vi "Read Value.vi"(8 "error in (no error)":errorcluster, 11 "Float D Element in":refnum<class "Float D Element.lvclass">) -> (0 "error out":errorcluster, 2 "Value":sgl, 3 "Float D Element out":refnum<class "Float D Element.lvclass">)   [LabVIEW 2018, in "D Datagrid Library.lvlib" / "Float D Element.lvclass"]
uses:
  Float D Element.lvclass
  Float D Element.lvclass/Float D Element.ctl
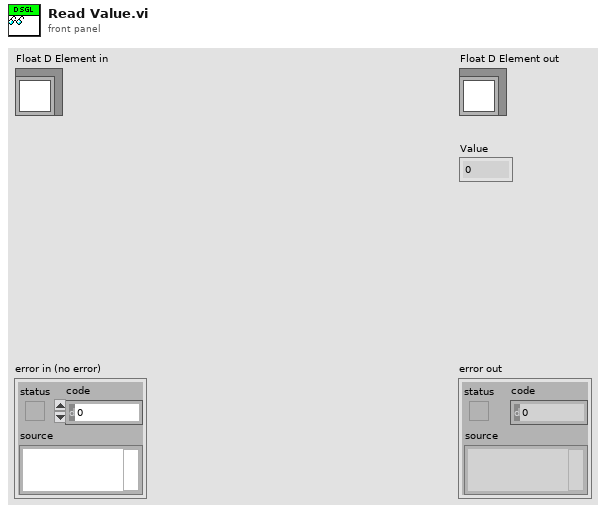
[diagram p1: front panel]
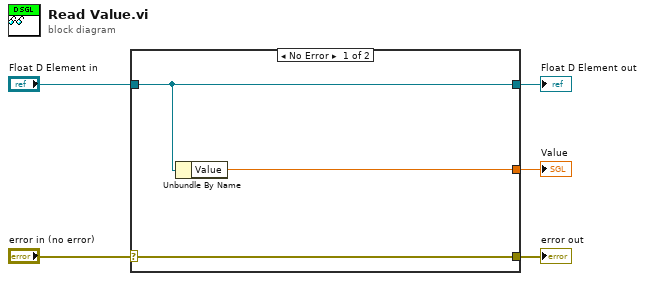
[diagram p0: block diagram]
diagram:
  n1 = case shown="No Error" "error in (no error)" {
    selector: "error in (no error)" -> [w8 w9]
    tunnel: [w8 w9] -> w4
    tunnel: [w7 w10] -> w2
    tunnel: "Float D Element in" -> [w7 w10]
    tunnel: [w6 _] -> w1
    frame No Error {
      n2 = Unbundle By Name(w7) -> ("Value"=w6:sgl)
    }
    frame Error {
    }
  }
  "error out" <- w4
  "Float D Element out" <- w2
  "Value" <- w1
